vi "ExecuteGrSimTest.vi"(6 "Replace Robots":bool, 7 "IA State Input":T3, 8 "Test Mode On":bool, 9 "reset":bool, 10 "id":i32, 11 "RandomPoints":dbl[][](array[numeric])) -> (1 "kick num":i32, 2 "Replace active":bool, 3 "grSim replacement":cluster{"robots":T1[], "ball":T2}={"robots"=[{"x"=0.0, "y"=-450.0, "dir"=0.0, "yellowteam"=FALSE, "id"=0}, {"x"=0.0, "y"=-270.0, "dir"=0.0, "yellowteam"=FALSE, "id"=1}, {"x"=0.0, "y"=-90.0, "dir"=0.0, "yellowteam"=FALSE, "id"=2}, {"x"=0.0, "y"=90.0, "dir"=0.0, "yellowteam"=FALSE, "id"=3}, {"x"=0.0, "y"=270.0, "dir"=0.0, "yellowteam"=FALSE, "id"=4}, {"x"=0.0, "y"=450.0, "dir"=0.0, "yellowteam"=FALSE, "id"=5}], "ball"={"x"=0.0, "y"=0.0, "vx"=0.0, "vy"=0.0}})   [LabVIEW 2017]
uses:
  Core/AI Input.ctl
  Core/AI Robot.ctl
  Intel/Functions Enum.ctl
  Intel/AttackerStates.ctl
  Path Planning/RRT/PathDests.ctl
  Path Planning/RRT/PathDest.ctl
  Core/AI Ball.ctl
  Core/Field Size.ctl
  Core/AI Judge.ctl
  Intel/Command Enum.ctl
  Util/Events/Events.ctl
  grSim RobotReplacement.ctl
  grSim_BallReplacement.ctl
panel:
  in  "Time":enum16{"Azul", "Amarelo"}(ring) caption="Enum"
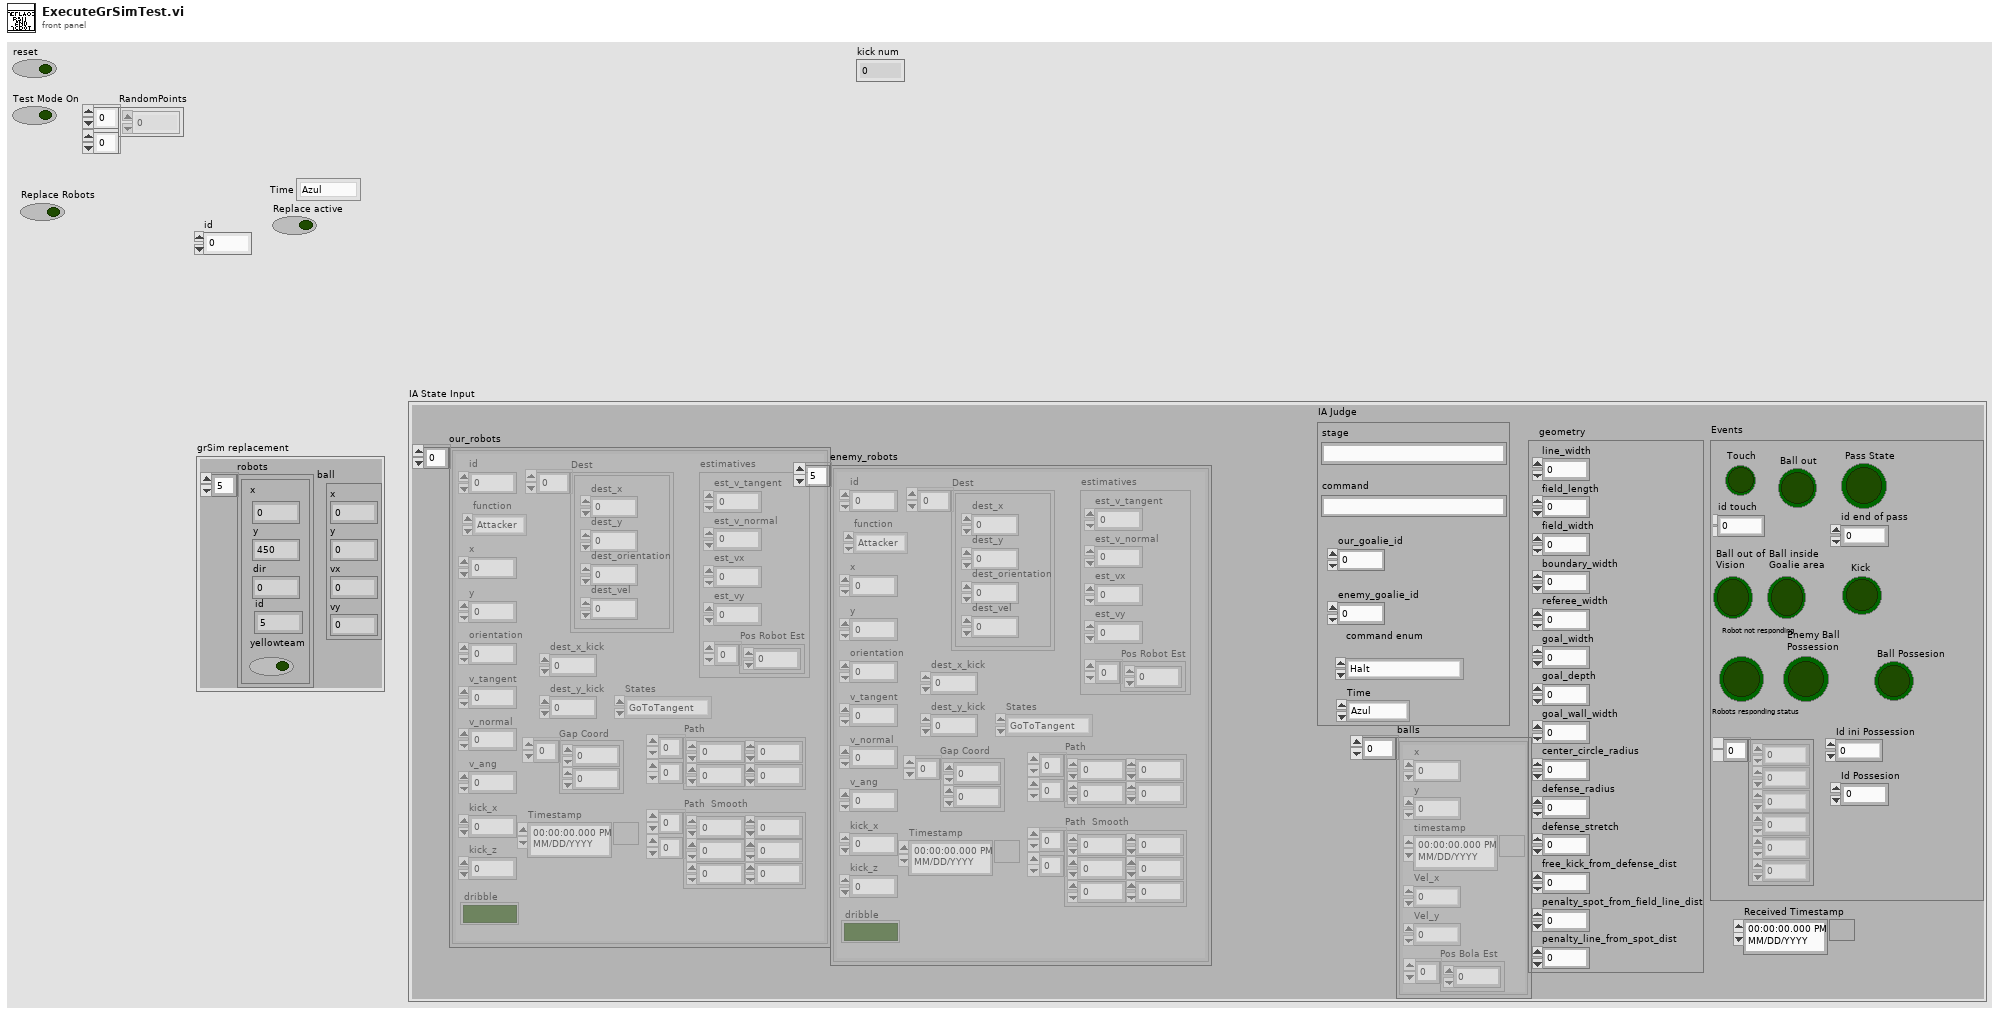
[diagram p1: front panel]
types:
  T1 = typedef "grSim RobotReplacement.ctl" = cluster{"x":dbl, "y":dbl, "dir":dbl, "yellowteam":bool, "id":u32}
  T2 = typedef "grSim_BallReplacement.ctl" = cluster{"x":dbl, "y":dbl, "vx":dbl, "vy":dbl}
  T3 = typedef "AI Input.ctl" = cluster{"our_robots":T4[], "enemy_robots":T4[], "balls":T9[], "geometry":T10, "IA Judge":T11, "Received Timestamp":timestamp, "Events":T13}
  T4 = typedef "AI Robot.ctl" = cluster{"id":u32, "function":T5, "x":dbl, "y":dbl, "orientation":dbl, "v_tangent":dbl, "v_normal":dbl, "v_ang":dbl, "kick_x":dbl, "kick_z":dbl, "dribble":bool, "Timestamp":timestamp, "estimatives":cluster{"est_v_tangent":dbl, "est_v_normal":dbl, "est_vx":dbl, "est_vy":dbl, "Pos Robot Est":dbl[]}, "dest_x_kick":dbl, "dest_y_kick":dbl, "Gap Coord":dbl[], "States":T6, "Path ":dbl[][], "Path  Smooth":dbl[][], "Dest":T7}
  T5 = typedef "Functions Enum.ctl" = enum16{"Attacker", "Goalie", "Defender", "Striker", "Goto 0", "Dummy", "Kicker", "ZigZag"}
  T6 = typedef "AttackerStates.ctl" = enum16{"Pass", "GoToTangent", "BallGetting", "GoToKick", ""}
  T7 = typedef "PathDests.ctl" = T8[]
  T8 = typedef "PathDest.ctl" = cluster{"dest_x":dbl, "dest_y":dbl, "dest_orientation":dbl, "dest_vel":dbl}
  T9 = typedef "AI Ball.ctl" = cluster{"x":dbl, "y":dbl, "timestamp":timestamp, "Vel_x":dbl, "Vel_y":dbl, "Pos Bola Est":dbl[]}
  T10 = typedef "Field Size.ctl" = cluster{"line_width":u32, "field_length":u32, "field_width":u32, "boundary_width":u32, "referee_width":u32, "goal_width":u32, "goal_depth":u32, "goal_wall_width":u32, "center_circle_radius":u32, "defense_radius":u32, "defense_stretch":u32, "free_kick_from_defense_dist":u32, "penalty_spot_from_field_line_dist":u32, "penalty_line_from_spot_dist":u32}
  T11 = typedef "AI Judge.ctl" = cluster{"stage":string, "command":string, "our_goalie_id":dbl, "enemy_goalie_id":dbl, "command enum":T12, "Time":enum16{"Azul", "Amarelo"}}
  T12 = typedef "Command Enum.ctl" = enum16{"Halt", "Stop", "Force Start", "PKA Normal Start", "Prepare Kickoff Ally", "PKE Normal Start", "Prepare Kickoff Enemy", "Prepare Penalty Ally", "PPA Normal Start", "Prepare Penalty Enemy", "PPE Normal Start", "Direct Free Enemy", "Direct Free Ally", "Indirect Free Enemy", "Indirect Free Ally", "Timeout Enemy", "Timeout Ally", "Goal Enemy", "Goal Ally", "Ball Placement Enemy", "Ball Placement Ally", "Normal Half Time", "Extra Time Break", "Extra Half Time", "None", "Post Game"}
  T13 = typedef "Events.ctl" = cluster{"Touch":bool, "Ball out":bool, "id touch":dbl, "Ball out of \nVision":bool, "Ball inside \nGoalie area":bool, "Robot not responding":bool, "Robots responding status":dbl[], "Enemy Ball \nPossession":bool, "Pass State":bool, "id end of pass":dbl, "Kick":bool, "Id ini Possession":dbl, "Ball Possesion":bool, "Id Possesion":dbl}
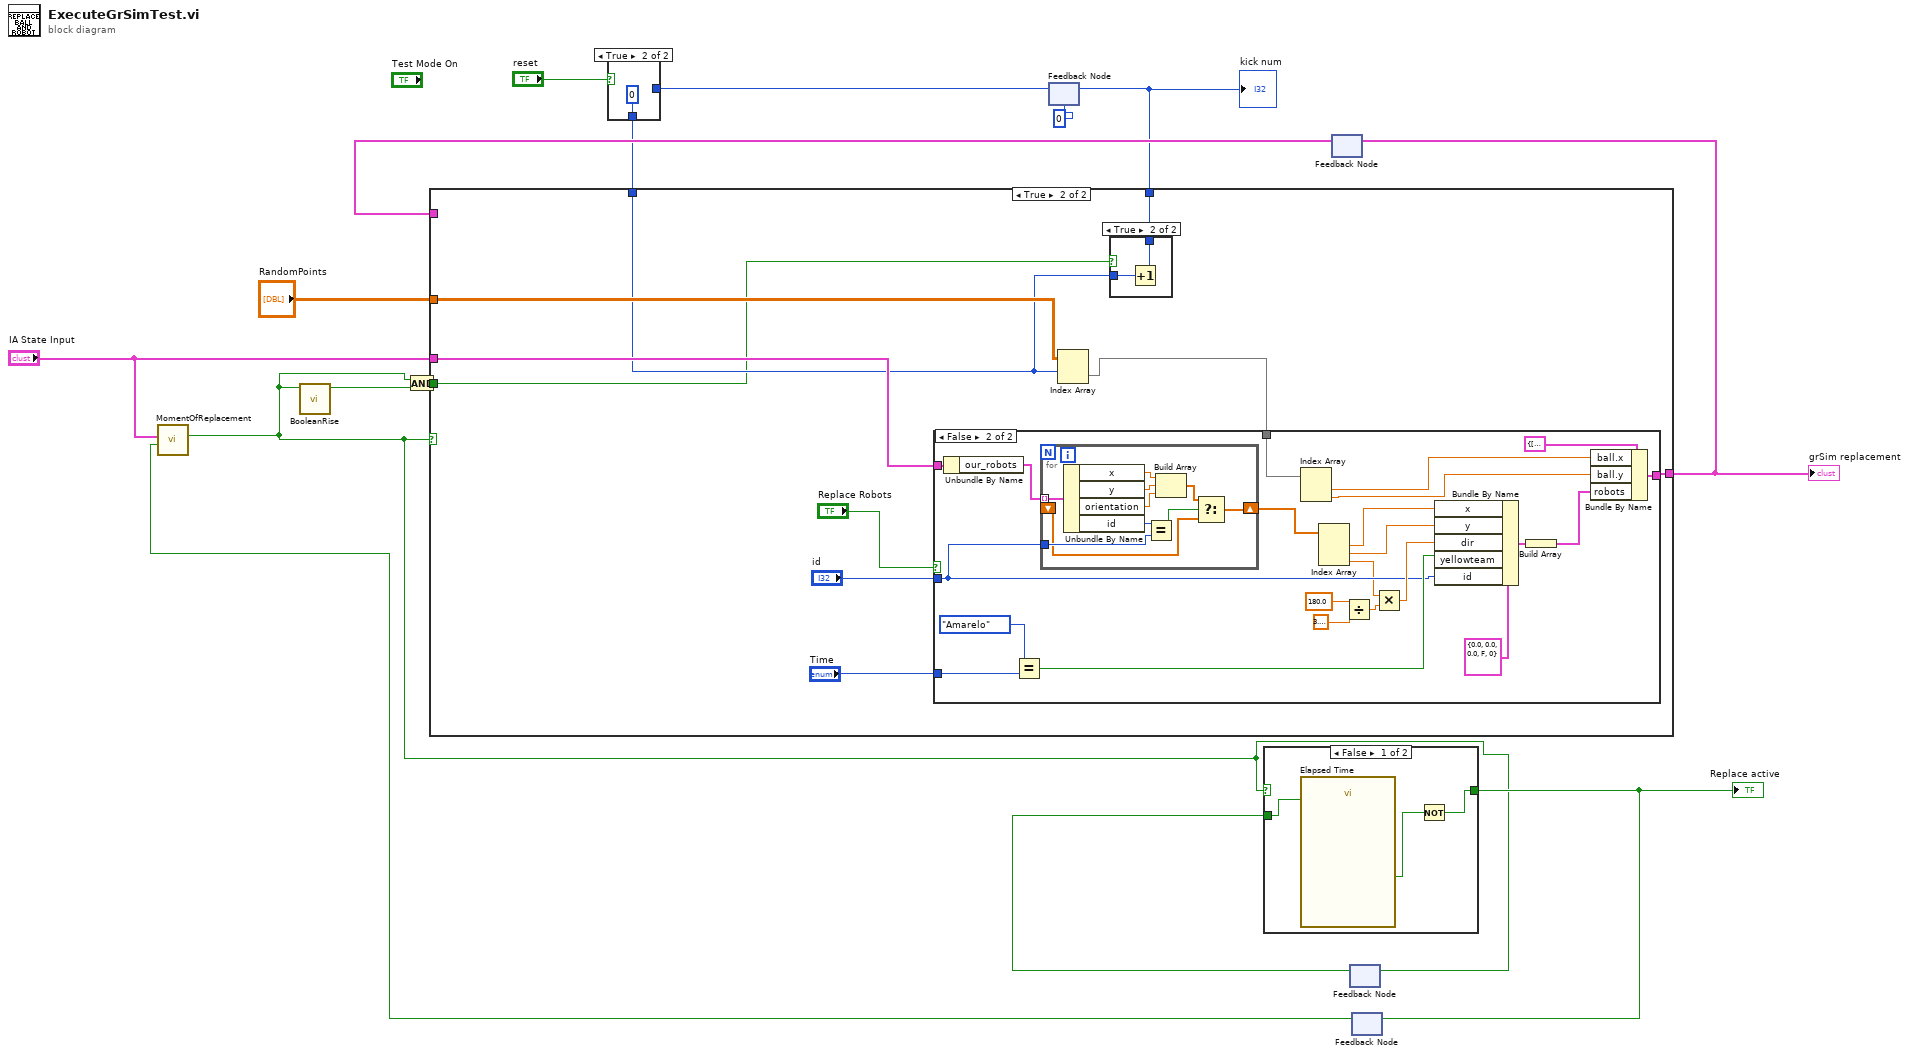
[diagram p0: block diagram]
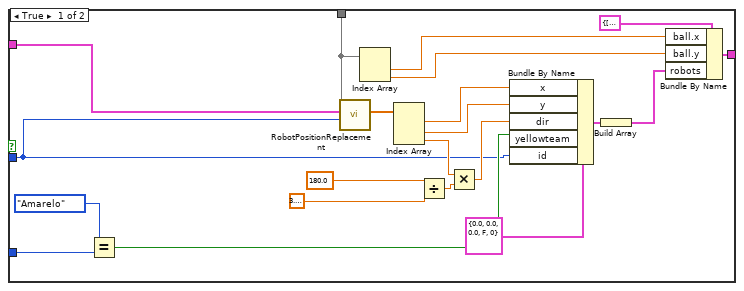
[diagram p6: hidden frame]
diagram:
  n1 = feedback #1(0) -> (w3:i32)
  n2 = case shown="True" "reset" {
    tunnel: w3 -> [w16 _]
    tunnel: [w16 0] -> w2
    frame False {
    }
    frame True {
    }
  }
  n3 = feedback #2() -> (w15:cluster{"robots":T1[], "ball":T2})  [unwired: 1 in]
  n4 = feedback #3() -> (w14:bool)  [unwired: 1 in]
  n5 = feedback #4() -> (w10:bool)  [unwired: 1 in]
  n6 = call "MomentOfReplacement.vi"("Replace active"=w10, "IA State Input"="IA State Input") -> ("Time to replace?"=w4:bool)  [unwired: 9 in]
  n7 = call "BooleanRise.vi"("Test Mode On"=w4) -> ("Boolean"=w5:bool)  [unwired: 10 in]
  n8 = And(x=w4, y=w5) -> (x .and. y?=w6:bool)
  n9 = case shown="True" w4 {
    tunnel: [w19 w29] -> w13
    tunnel: "IA State Input" -> [_ w26]
    tunnel: w15 -> [w19 _]
    tunnel: "RandomPoints" -> [_ w25]
    tunnel: w2 -> [w18 w22]
    tunnel: [w18 w21] -> w7
    tunnel: w6 -> [_ w20]
    frame False {
    }
    frame True {
      n10 = Index Array(array=w25, index (row)=w22) -> (element=w28:dbl[])  [unwired: 1 in]
      n11 = case shown="False" "Replace Robots" {
        tunnel: [w53 w75] -> w29
        tunnel: w28 -> [w36 w57]
        tunnel: "Time" -> [w49 w71]
        tunnel: w26 -> [w44 w64]
        tunnel: "id" -> [w37 w62]
        frame True {
          n12 = Equal?(x=enum16{"Azul", "Amarelo"}."Amarelo", y=w49) -> (x = y?=w47:bool)
          n13 = call "RobotPositionReplacement.vi"("id"=w37, "IA State Input"=w44, "Position Ball"=w36) -> ("Position Robot"=w46:dbl[])  [unwired: 6 in]
          n14 = Index Array(array=w36) -> (element #1=w35:dbl, element #2=w34:dbl)  [unwired: 2 in]
          n15 = Index Array(array=w46) -> (element #1=w45:dbl, element #2=w43:dbl, element #3=w38:dbl)  [unwired: 3 in]
          n16 = Divide(x=180.0, y=3.141592653589793) -> (x/y=w41:dbl)
          n17 = Multiply(x=w38, y=w41) -> (x*y=w42:dbl)
          n18 = Bundle By Name(cluster=T1 {"x"=0.0, "y"=0.0, "dir"=0.0, "yellowteam"=FALSE, "id"=0} ("element"), "x"=w45, "y"=w43, "dir"=w42, "yellowteam"=w47, "id"=w37) -> (w51:T1)
          n19 = Build Array(w51) -> (w50:T1[])
          n20 = Bundle By Name(cluster=cluster{"robots":T1[], "ball":T2} {"robots"=[{"x"=0.0, "y"=-450.0, "dir"=0.0, "yellowteam"=FALSE, "id"=0}, {"x"=0.0, "y"=-270.0, "dir"=0.0, "yellowteam"=FALSE, "id"=1}, {"x"=0.0, "y"=-90.0, "dir"=0.0, "yellowteam"=FALSE, "id"=2}, {"x"=0.0, "y"=90.0, "dir"=0.0, "yellowteam"=FALSE, "id"=3}, {"x"=0.0, "y"=270.0, "dir"=0.0, "yellowteam"=FALSE, "id"=4}, {"x"=0.0, "y"=450.0, "dir"=0.0, "yellowteam"=FALSE, "id"=5}], "ball"={"x"=0.0, "y"=0.0, "vx"=0.0, "vy"=0.0}} ("grSim replacement"), "ball.x"=w35, "ball.y"=w34, "robots"=w50) -> (w53:cluster{"robots":T1[], "ball":T2})
        }
        frame False {
          n21 = Unbundle By Name(w64) -> ("our_robots"=w63:T4[])
          n22 = Equal?(x=enum16{"Azul", "Amarelo"}."Amarelo", y=w71) -> (x = y?=w69:bool)
          n23 = for {
            tunnel: w63 -> [w85] mode=indexing
            tunnel: w62 -> [w83]
            shift-right: [w77] -> w61
            shift-left: _ -> [w76]
            n24 = Unbundle By Name(w85) -> ("x"=w82:dbl, "y"=w81:dbl, "orientation"=w80:dbl, "id"=w84:u32)
            n25 = Equal?(x=w84, y=w83) -> (x = y?=w79:bool)
            n26 = Build Array(w82, w81, w80) -> (w78:dbl[])
            n27 = Select(t=w78, s=w79, f=w76) -> (s? t:f=w77:dbl[])
          }
          n28 = Index Array(array=w57) -> (element #1=w56:dbl, element #2=w55:dbl)  [unwired: 2 in]
          n29 = Index Array(array=w61) -> (element #1=w60:dbl, element #2=w58:dbl, element #3=w59:dbl)  [unwired: 3 in]
          n30 = Divide(x=180.0, y=3.141592653589793) -> (x/y=w67:dbl)
          n31 = Multiply(x=w59, y=w67) -> (x*y=w68:dbl)
          n32 = Bundle By Name(cluster=T1 {"x"=0.0, "y"=0.0, "dir"=0.0, "yellowteam"=FALSE, "id"=0} ("element"), "x"=w60, "y"=w58, "dir"=w68, "yellowteam"=w69, "id"=w62) -> (w73:T1)
          n33 = Build Array(w73) -> (w72:T1[])
          n34 = Bundle By Name(cluster=cluster{"robots":T1[], "ball":T2} {"robots"=[{"x"=0.0, "y"=-450.0, "dir"=0.0, "yellowteam"=FALSE, "id"=0}, {"x"=0.0, "y"=-270.0, "dir"=0.0, "yellowteam"=FALSE, "id"=1}, {"x"=0.0, "y"=-90.0, "dir"=0.0, "yellowteam"=FALSE, "id"=2}, {"x"=0.0, "y"=90.0, "dir"=0.0, "yellowteam"=FALSE, "id"=3}, {"x"=0.0, "y"=270.0, "dir"=0.0, "yellowteam"=FALSE, "id"=4}, {"x"=0.0, "y"=450.0, "dir"=0.0, "yellowteam"=FALSE, "id"=5}], "ball"={"x"=0.0, "y"=0.0, "vx"=0.0, "vy"=0.0}} ("grSim replacement"), "ball.x"=w56, "ball.y"=w55, "robots"=w72) -> (w75:cluster{"robots":T1[], "ball":T2})
        }
      }
      n35 = case shown="True" w20 {
        tunnel: w22 -> [w30 w32]
        tunnel: [w30 w31] -> w21
        frame False {
        }
        frame True {
          n36 = Increment(x=w32) -> (x+1=w31:i32)
        }
      }
    }
  }
  "grSim replacement" <- w13
  "kick num" <- w7
  n37 = feedback-in #1(w7) -> ()
  n38 = case shown="False" w4 {
    selector: w4 -> [_ w89]
    tunnel: [w88 w89] -> w11
    tunnel: w14 -> [w86 _]
    frame False {
      n39 = call "Elapsed Time"("Reset"=w86) -> ("Time has Elapsed"=w87:bool)  [unwired: 11 in, 7 out]
      n40 = Not(x=w87) -> (.not. x?=w88:bool)
    }
    frame True {
    }
  }
  "Replace active" <- w11
  n41 = feedback-in #2(w13) -> ()
  n42 = feedback-in #3(w4) -> ()
  n43 = feedback-in #4(w11) -> ()
